vi "NI VeriStand - Get Alarms Status.vi"(7 "Target":string, 8 "error in (no error)":errorcluster, 11 "AlarmManager in":T1) -> (0 "error out":errorcluster, 1 "Active High Alarm":string, 2 "Status":cluster{"High":bool, "Medium":bool, "Low":bool}, 3 "AlarmManager out":T1, 4 "Active Medium Alarm":string, 6 "Active Low Alarm":string)   [LabVIEW 2020, in "NI_VS AlarmManager ExecutionAPI.lvlib"]
uses:
  <vilib>/NI VeriStand/Execution/AlarmManager/NI_VS AlarmManager ExecutionAPI.lvlib
  <vilib>/NI VeriStand/Execution/AlarmManager/AlarmManagerAPI.ctl
  NationalInstruments.VeriStand.ClientAPI
panel:
  # "Obsolete. Strict priorities of low, medium, and high are no longer supported. Valid priorities now range from 0 - 31. This function will only test alarms in group 0.\n\nUse Get Alarm Multiple Alarms\nData.vi or Get Alarm Data.vi"
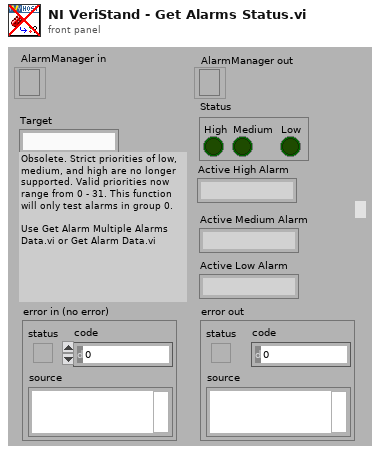
[diagram p1: front panel]
types:
  T1 = typedef "NI_VS AlarmManager ExecutionAPI.lvlib/AlarmManagerAPI.ctl" = refnum<k24>
  T2 = cluster{"highAlarm":bool, "medAlarm":bool, "lowAlarm":bool}
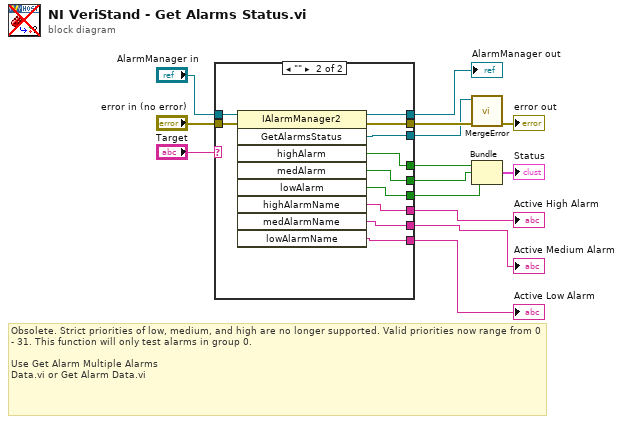
[diagram p0: block diagram]
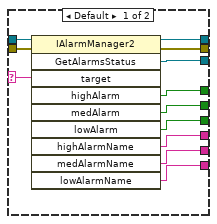
[diagram p2: hidden frame]
diagram:
  # "Obsolete. Strict priorities of low, medium, and high are no longer supported. Valid priorities now range from 0 - 31. This function will only test alarms in group 0.\n\nUse Get Alarm Multiple Alarms\nData.vi or Get Alarm Data.vi"
  n1 = case shown="\"\"" "Target" {
    selector: "Target" -> [w15 _]
    tunnel: "AlarmManager in" -> [w26 w37]
    tunnel: [w25 w36] -> w13
    tunnel: [w24 w35] -> w12
    tunnel: [w23 w34] -> w11
    tunnel: "error in (no error)" -> [w22 w33]
    tunnel: [w21 w32] -> w7
    tunnel: [w20 w31] -> w6
    tunnel: [w19 w30] -> w5
    tunnel: [w18 w29] -> w4
    tunnel: [w17 w28] -> w3
    tunnel: [w16 w27] -> w2
    frame Default {
      n2 = invoke class="IAlarmManager2" method="GetAlarmsStatus"(reference=w26, error in=w22, "target"=w15) -> (reference out=w25:T1, error out=w24:errorcluster, "GetAlarmsStatus"=w23:refnum<k24>, "highAlarm"=w21:bool, "medAlarm"=w20:bool, "lowAlarm"=w19:bool, "highAlarmName"=w18:string, "medAlarmName"=w17:string, "lowAlarmName"=w16:string)  [unwired: 7 in, 1 out]
    }
    frame "" {
      n3 = invoke class="IAlarmManager2" method="GetAlarmsStatus"(reference=w37, error in=w33) -> (reference out=w36:T1, error out=w35:errorcluster, "GetAlarmsStatus"=w34:refnum<k24>, "highAlarm"=w32:bool, "medAlarm"=w31:bool, "lowAlarm"=w30:bool, "highAlarmName"=w29:string, "medAlarmName"=w28:string, "lowAlarmName"=w27:string)  [unwired: 7 in]
    }
  }
  "AlarmManager out" <- w13
  "Active High Alarm" <- w4
  "Active Medium Alarm" <- w3
  "Active Low Alarm" <- w2
  n4 = call <vilib>:"MergeError.vi"("error in (no error)"=w12, "Error"=w11) -> ("error out"=→"error out":errorcluster)  [unwired: 9 out]
  n5 = Bundle("highAlarm"=w7, "medAlarm"=w6, "lowAlarm"=w5) -> (→"Status":T2)  [unwired: 1 out]
